vi "Configure_Indexes.vi"() -> ()   [LabVIEW 2018]
uses:
  <vilib>/robotics/Steering/Wheel/Rotation Direction.ctl
  <vilib>/robotics/Steering/Wheel/Wheel Parameters.ctl
  <vilib>/Studica/Studica Toolkit/Background/Mxp Selection.ctl
  <vilib>/robotics/Steering/Omnidirectional Wheel/NI_Robotics_Omnidirectional Wheel.lvclass
  C:/Program Files (x86)/National Instruments/LabVIEW 2018/vi.lib/robotics/Steering/Wheel/NI_Robotics_Wheel.lvclass
  <vilib>/robotics/Steering/Omnidirectional Wheel/Create Omnidirectional Wheel.vi
  <vilib>/robotics/Steering/Steering Frame/Create User Defined Steering Frame.vi
  <vilib>/robotics/Steering/Steering Frame/Apply Steering Frame Velocity to Motors.vi
  <vilib>/robotics/Steering/Wheel/NI_Robotics_Wheel.lvclass
  <vilib>/robotics/Steering/Steering Frame/NI_Robotics_Steering Frame.lvclass
panel:
  in  "theta":dbl
  in  "y":dbl
  in  "x":dbl
  in  "Reset Encoders":bool
  out "Actual-SpeedList":dbl[](array[numeric])
  out "Tick Count(uSec)":u32 caption="Tick Count(Ticks)"
  out "ccw motor velocity setpoints":dbl[](array[numeric])
  in  "wheel indexes":i32[](array[numeric])
  in  "stop":bool
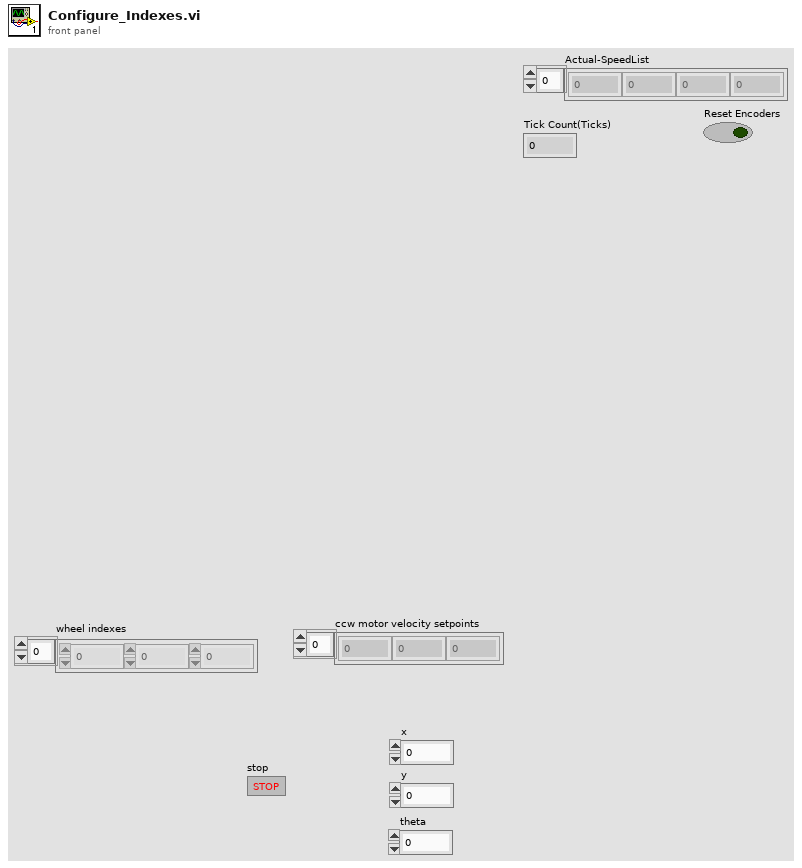
[diagram p1: front panel]
types:
  T1 = typedef "Mxp Selection.ctl" = enum16{"MXP A", "MXP B"}
  T2 = typedef "NI_Robotics_Wheel.lvclass/Wheel Parameters.ctl" = cluster{"wheel radius":dbl, "gear ratio":dbl, "forward rotation direction":T3}
  T3 = typedef "NI_Robotics_Wheel.lvclass/Rotation Direction.ctl" = u16
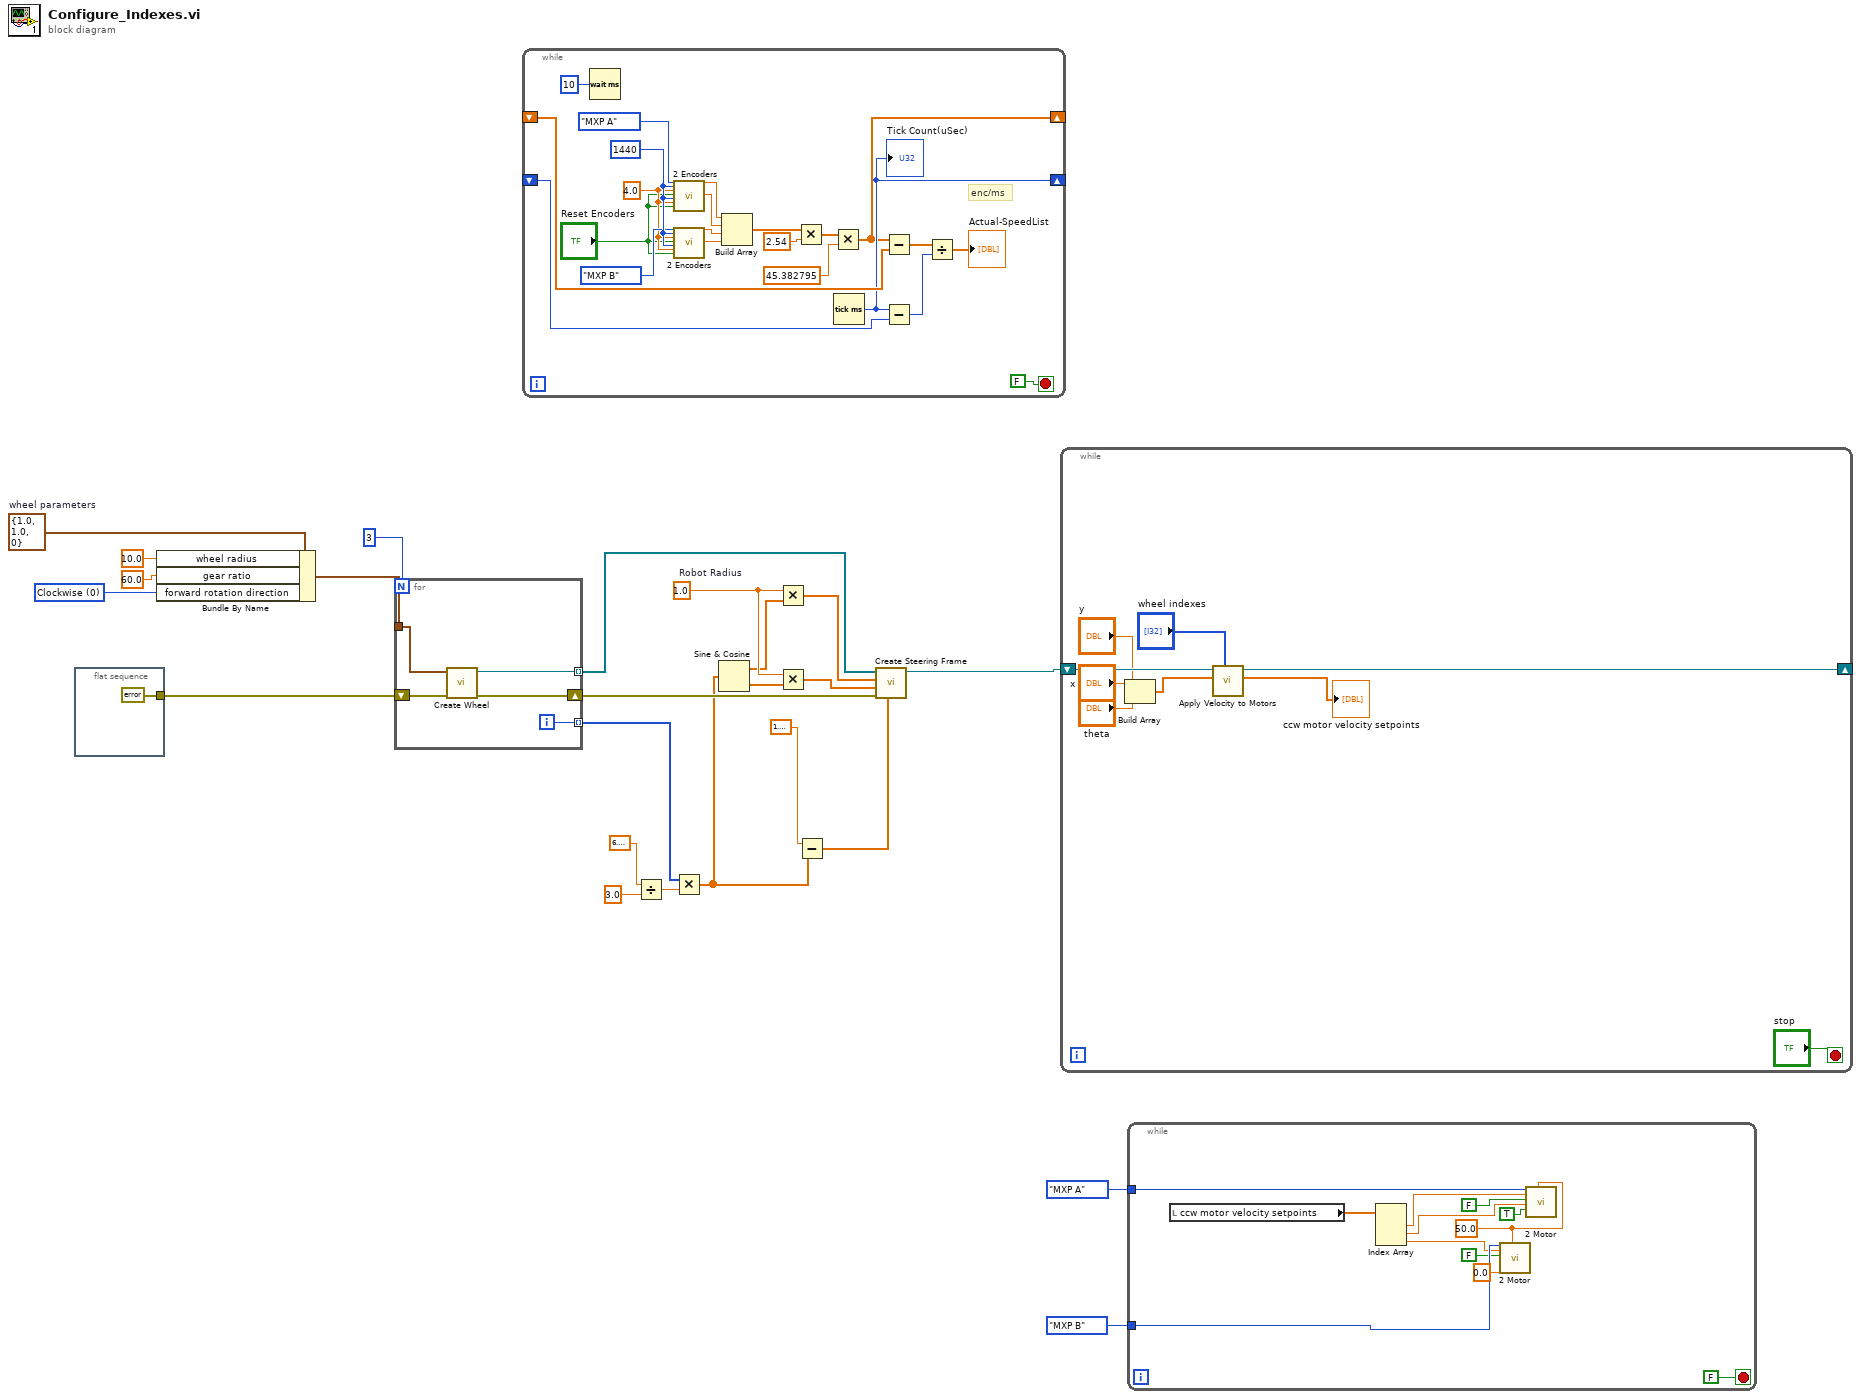
[diagram p0: block diagram]
diagram:
  w24 = T2 {"wheel radius"=1.0, "gear ratio"=1.0, "forward rotation direction"=0}  # wheel parameters
  w9 = T3 0 items=["Clockwise", "Counterclockwise"] ("forward rotation direction")
  w14 = 1.0  # Robot Radius
  n1 = flat-sequence {
    tunnel: [errorcluster {"status"=FALSE, "code"=0, "source"=""} ("error out")] -> w20
    frame #0 {
    }
  }
  n2 = Bundle By Name(cluster=w24, "wheel radius"=10.0, "gear ratio"=60.0, "forward rotation direction"=w9) -> (w21:T2)
  n3 = for {
    N: 3 -> [_]
    shift-right: [w29] -> w7
    shift-left: w20 -> [w30]
    tunnel: [w28] -> w19 mode=indexing
    tunnel: w21 -> [w27]
    tunnel: [w26] -> w15 mode=indexing
    i -> [w26]
    n4 = call-poly <vilib>:"Create Wheel.vi"("error in (no error)"=w30, "wheel parameters"=w27) -> ("error out"=w29:errorcluster, "omni wheel out"=w28:refnum<class "NI_Robotics_Omnidirectional Wheel.lvclass">)  [unwired: 8 in]
  }
  n5 = while {
    shift-right: [w35] -> _
    shift-left: _ -> [w40]
    shift-right: [w36] -> _
    shift-left: _ -> [w38]
    stop <- FALSE stop-if-true
    w32 = 4.0 ("Wheel Diameter M1 (inches)")
    w43 = u32 1440 ("Ticks Per Rev M0")
    # "enc/ms"
    n6 = Wait (ms)(milliseconds to wait=u32 10) -> ()  [unwired: 1 out]
    n7 = call <vilib>:"2 Encoders.vi"("Mxp Side"=Mxp_Selection."MXP A", "Ticks Per Rev M0"=w43, "Wheel Diameter M0 (inches)"=w32, "Reset Encoder 0"="Reset Encoders", "Ticks Per Rev M1"=w43, "Wheel Diameter M1 (inches)"=w32, "Reset Encoder 1"="Reset Encoders") -> ("Distance M0 (inches)"=w44:dbl, "Distance M1 (inches)"=w45:dbl)  [unwired: 18 in, 1 out]
    n8 = call <vilib>:"2 Encoders.vi"("Mxp Side"=Mxp_Selection."MXP B", "Ticks Per Rev M0"=w43, "Wheel Diameter M0 (inches)"=w32, "Reset Encoder 0"="Reset Encoders", "Ticks Per Rev M1"=w43, "Wheel Diameter M1 (inches)"=w32, "Reset Encoder 1"="Reset Encoders") -> ("Distance M0 (inches)"=w46:dbl, "Distance M1 (inches)"=w33:dbl)  [unwired: 18 in, 1 out]
    n9 = Build Array(w44, w45, w46, w33) -> (w48:dbl[])
    n10 = Multiply(x=w48, y=2.54) -> (x*y=w49:dbl[])
    n11 = Multiply(x=w49, y=45.382795) -> (x*y=w35:dbl[])
    n12 = Tick Count (ms)() -> (millisecond timer value=w36:u32)
    "Tick Count(uSec)" <- w36
    n13 = Subtract(x=w35, y=w40) -> (x-y=w39:dbl[])
    n14 = Subtract(x=w36, y=w38) -> (x-y=w51:u32)
    n15 = Divide(x=w39, y=w51) -> (x/y=→"Actual-SpeedList":dbl[])
  }
  n16 = Divide(x=6.283185307179586, y=3.0) -> (x/y=w16:dbl)
  n17 = Multiply(x=w15, y=w16) -> (x*y=w4:dbl[])
  n18 = Sine & Cosine(0:w4) -> (1:w6:dbl[], 2:w5:dbl[])
  n19 = Multiply(x=w14, y=w6) -> (x*y=w13:dbl[])
  n20 = Multiply(x=w14, y=w5) -> (x*y=w12:dbl[])
  n21 = Subtract(x=1.5707963267948966, y=w4) -> (x-y=w10:dbl[])
  n22 = call-poly <vilib>:"Create Steering Frame.vi"("wheel frame angles (rad)"=w10, "error in (no error)"=w7, "wheel y positions"=w12, "wheel x positions"=w13, "wheels"=w19) -> ("steering frame out"=w3:refnum<class "NI_Robotics_Steering Frame.lvclass">)  [unwired: 5 in, 1 out]
  n23 = while {
    shift-right: [w59] -> _
    shift-left: w3 -> [w60]
    stop <- "stop" stop-if-true
    n24 = Build Array("x", "y", "theta") -> (w57:dbl[])
    n25 = call-poly <vilib>:"Apply Velocity to Motors.vi"("wheel indexes"="wheel indexes", "steering frame velocity"=w57, "steering frame in"=w60) -> ("ccw motor velocity setpoints"=→"ccw motor velocity setpoints":dbl[], "steering frame out"=w59:refnum<class "NI_Robotics_Steering Frame.lvclass">)  [unwired: 4 in, 3 out]
  }
  n26 = while {
    tunnel: Mxp_Selection."MXP A" ("Mxp Side") -> [w73]
    tunnel: Mxp_Selection."MXP B" ("Mxp Side") -> [w72]
    stop <- FALSE stop-if-true
    w70 = 50.0 ("Frequency [Hz]")
    n27 = local read "ccw motor velocity setpoints"() -> (w71:dbl[])
    n28 = Index Array(array=w71) -> (element #1=w66:dbl, element #2=w65:dbl, element #3=w64:dbl)  [unwired: 3 in]
    n29 = call <vilib>:"2 Motor.vi"("Mxp Side"=w72, "Speed M0"=w64, "Invert M0"=FALSE, "Speed M1"=0.0, "Frequency [Hz]"=w70) -> ()  [unwired: 14 in, 1 out]
    n30 = call <vilib>:"2 Motor.vi"("Mxp Side"=w73, "Speed M0"=w66, "Invert M0"=FALSE, "Speed M1"=w65, "Invert M1"=TRUE ("Invert M0"), "Frequency [Hz]"=w70) -> ()  [unwired: 13 in, 1 out]
  }
